vi "Read Limit Tests.vi"(0 "VISA resource name":refnum<visa-resource-name>, 11 "error in (no error)":errorcluster) -> (4 "VISA resource name out":refnum<visa-resource-name>, 6 "Limit1 Test Failed":bool, 8 "Limit2 Test Failed":bool, 15 "error out":errorcluster)   [LabVIEW 2011, in "Keithley 2182.lvlib"]
doc: "Performs and reads the two limit tests.\n\n\n<B>Note:</B>\nYou must first configure Limit Tests using <B>Configure Limit Test</B> VI."
uses:
  Keithley 2182.lvlib
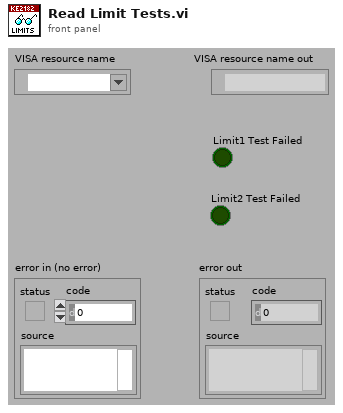
[diagram p1: front panel]
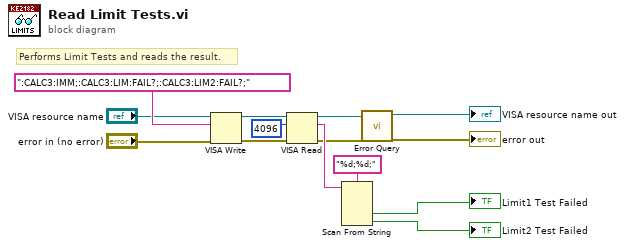
[diagram p0: block diagram]
diagram:
  # "Performs Limit Tests and reads the result."
  n1 = VISA Write(VISA resource name="VISA resource name", write buffer=":CALC3:IMM;:CALC3:LIM:FAIL?;:CALC3:LIM2:FAIL?;", error in (no error)="error in (no error)") -> (VISA resource name out=w11:refnum<visa-resource-name>, error out=w12:errorcluster)  [unwired: 1 out]
  n2 = VISA Read(VISA resource name=w11, byte count=u32 4096, error in (no error)=w12) -> (VISA resource name out=w5:refnum<visa-resource-name>, read buffer=w7:string, error out=w6:errorcluster)  [unwired: 1 out]
  n3 = Scan From String(format string="%d;%d;", input string=w7) -> (output 1=→"Limit1 Test Failed":bool, output 2=→"Limit2 Test Failed":bool)  [unwired: 4 in, 3 out]
  n4 = call "Error Query.vi"("error in (no error)"=w6, "VISA resource name"=w5) -> ("error out"=→"error out":errorcluster, "VISA resource name out"=→"VISA resource name out":refnum<visa-resource-name>)  [unwired: 6 in, 2 out]
